vi "PruebaAutoRefresh.vi"() -> ()   [LabVIEW 2014, in "MSX-E3701.lvlib"]
uses:
  MSX-E3701.lvlib
  DriverMasterSync/build/DriverMasterSync.lvlibp/APIs/Data Queue/Control Data Cluster.ctl
  DriverMasterSync/build/DriverMasterSync.lvlibp/APIs/Data Queue/Acquisition Data 1 Sample Cluster.ctl
  DriverMasterSync/build/DriverMasterSync.lvlibp/Modules/HAL/TypeDefs/HAL Config Data.ctl
  MSX-E3701Class/MSX-E3701.lvclass
  DriverMasterSync/build/DriverMasterSync.lvlibp/APIs/Data Queue/WINFAS 2 Data Queue.lvlib
  DriverMasterSync/build/DriverMasterSync.lvlibp
panel:
  in  "PromCycle":bool
  out "HAL Config Data":T1
  out "1 Sample":T2
  out "Control Data":T3
  in  "stop":bool
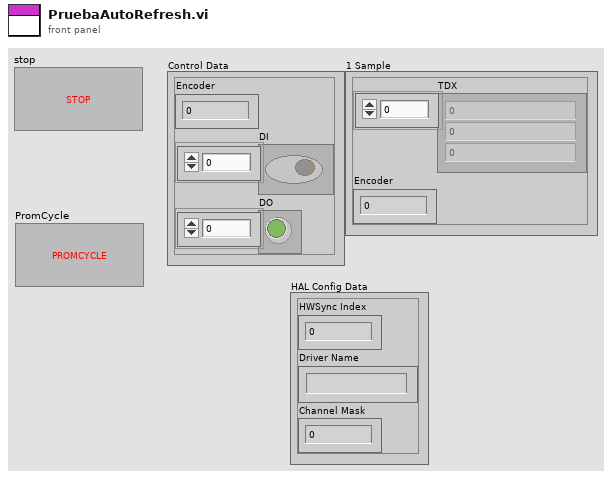
[diagram p1: front panel]
types:
  T1 = typedef "DriverMasterSync.lvlibp/HAL Config Data.ctl" = cluster{"HWSync Index":u32, "Driver Name":string, "Channel Mask":u64}
  T2 = typedef "DriverMasterSync.lvlibp/WINFAS 2 Data Queue.lvlib/Acquisition Data 1 Sample Cluster.ctl" = cluster{"TDX":sgl[], "Encoder":sgl}
  T3 = typedef "DriverMasterSync.lvlibp/WINFAS 2 Data Queue.lvlib/Control Data Cluster.ctl" = cluster{"Encoder":sgl, "DI":bool[], "DO":bool[]}
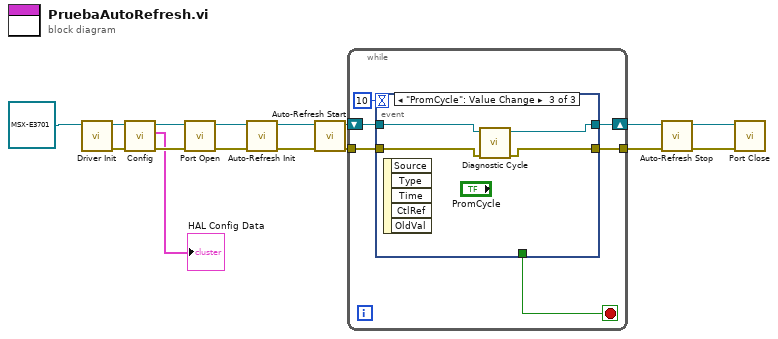
[diagram p0: block diagram]
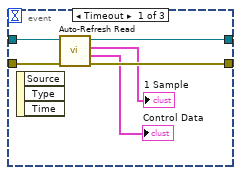
[diagram p2: hidden frame]
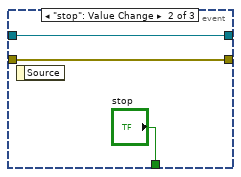
[diagram p3: hidden frame]
diagram:
  n1 = call-dynamic "Driver Init.vi"("MSX-E3701 in"=refnum<class "MSX-E3701.lvclass"> refnum) -> ("error out"=w7:errorcluster, "MSX-E3701 out"=w8:refnum<class "MSX-E3701.lvclass">)  [unwired: 9 in]
  n2 = call-dynamic "Config.vi"("error in (no error)"=w7, "MSX-E3701 in"=w8) -> ("error out"=w12:errorcluster, "HAL Config Data"=→"HAL Config Data":T1, "MSX-E3701 out"=w16:refnum<class "MSX-E3701.lvclass">)  [unwired: 7 in]
  n3 = call-dynamic "Port Open.vi"("error in (no error)"=w12, "MSX-E3701 in"=w16) -> ("error out"=w11:errorcluster, "MSX-E3701 out"=w15:refnum<class "MSX-E3701.lvclass">)  [unwired: 8 in]
  n4 = call-dynamic "Auto-Refresh Init.vi"("error in (no error)"=w11, "MSX-E3701 in"=w15) -> ("error out"=w10:errorcluster, "MSX-E3701 out"=w14:refnum<class "MSX-E3701.lvclass">)  [unwired: 8 in]
  n5 = call-dynamic "Auto-Refresh Start.vi"("error in (no error)"=w10, "MSX-E3701 in"=w14) -> ("error out"=w3:errorcluster, "MSX-E3701 out"=w4:refnum<class "MSX-E3701.lvclass">)  [unwired: 8 in]
  n6 = while {
    tunnel: w3 -> [w21]
    tunnel: [w19] -> w1
    shift-right: [w20] -> w2
    shift-left: w4 -> [w22]
    stop <- w18 stop-if-true
    n7 = event shown="[2] \"PromCycle\": Value Change" {
      selector: _ -> [_ _ _]
      dyn-events: _ -> [_ _ _]
      timeout: 10 -> [_ _ _]
      tunnel: w22 -> [w28 w29 w33]
      tunnel: w21 -> [w27 w30 w32]
      tunnel: [w26 w29 w35] -> w20
      tunnel: [w25 w30 w34] -> w19
      tunnel: [_ "stop" _] -> w18
      event Timeout {
        n8 = event-data() -> ()  [unwired: 1 in, 3 out]
        n9 = call-dynamic "Auto-Refresh Read.vi"("error in (no error)"=w27, "MSX-E3701 in"=w28) -> ("error out"=w25:errorcluster, "Control Data"=→"Control Data":T3, "1 Sample"=→"1 Sample":T2, "MSX-E3701 out"=w26:refnum<class "MSX-E3701.lvclass">)  [unwired: 6 in]
      }
      event "stop": Value Change {
        n10 = event-data() -> ()  [unwired: 1 in, 1 out]
      }
      event "PromCycle": Value Change {
        n11 = event-data() -> ()  [unwired: 1 in, 5 out]
        n12 = call-dynamic "Diagnostic Cycle.vi"("error in (no error)"=w32, "MSX-E3701 in"=w33) -> ("error out"=w34:errorcluster, "MSX-E3701 out"=w35:refnum<class "MSX-E3701.lvclass">)  [unwired: 8 in]
      }
    }
  }
  n13 = call-dynamic "Auto-Refresh Stop.vi"("error in (no error)"=w1, "MSX-E3701 in"=w2) -> ("error out"=w9:errorcluster, "MSX-E3701 out"=w13:refnum<class "MSX-E3701.lvclass">)  [unwired: 8 in]
  n14 = call-dynamic "Port Close.vi"("error in (no error)"=w9, "MSX-E3701 in"=w13) -> ()  [unwired: 8 in, 2 out]
